vi "Allocate Staff.vi"(0 "Room Service Monitor Model in":refnum<class "Room Service Monitor Model.lvclass">, 5 "Staff Name":string[](array[string]), 11 "error in (no error)":errorcluster) -> (4 "Room Service Monitor Model out":refnum<class "Room Service Monitor Model.lvclass">, 15 "error out":errorcluster)   [LabVIEW 2023, in "Room Service Monitor Model.lvlib" / "Room Service Monitor Model.lvclass"]
uses:
  Room Service Monitor Model.lvclass
  C:/Program Files/National Instruments/LabVIEW 2023/vi.lib/ActorFramework/Actor/Actor.lvclass
  <vilib>/ActorFramework/Actor/Actor.lvclass/Actor.ctl
  <vilib>/ActorFramework/Message Enqueuer/Message Enqueuer.lvclass/Message Enqueuer.ctl
  Room Service Monitor Model.lvclass/Room Service Monitor Model.ctl
  Room Service Monitor Model Messages/Launch Service Monitor Msg/Launch Service Monitor Msg.lvclass/Launch Service Monitor Msg.ctl
  Interfaces/Incoming Hotel Management Tool Model Interface Messages/Update Staff Allocation Msg/Update Staff Allocation Msg.lvclass/Update Staff Allocation Msg.ctl
  <vilib>/ActorFramework/Message Enqueuer/Init from Existing Queue.vi
  <vilib>/ActorFramework/Message Enqueuer/Enqueue.vi
  Room Service Monitor Model Messages/Launch Service Monitor Msg/Launch Service Monitor Msg.lvclass
  C:/Program Files/National Instruments/LabVIEW 2023/vi.lib/ActorFramework/Message/Message.lvclass
  Interfaces/Incoming Hotel Management Tool Model Interface Messages/Update Staff Allocation Msg/Update Staff Allocation Msg.lvclass
  Room Service Monitor Model Messages/Check Staff Msg/Check Staff Msg.lvclass
  <vilib>/ActorFramework/Message Priority Queue/Priority Enqueue.vi
  <vilib>/ActorFramework/Message Enqueuer/Message Enqueuer.lvclass
  Room Service Types/Room Service Base/Room Service Base.lvclass
  <vilib>/ActorFramework/Actor/Actor.lvclass
  C:/Users/bhaghyaraj/Trainings/NI Actor Framework/SDLC/Model Base/Model Base/Model Base.lvclass
  C:/Users/bhaghyaraj/Trainings/NI Actor Framework/SDLC/Interfaces/Model Base/Incoming Model Base Interface.lvclass
  C:/Users/bhaghyaraj/Trainings/NI Actor Framework/SDLC/Room Service Monitor Model/Room Service Monitor Model/Room Service Monitor Model.lvclass
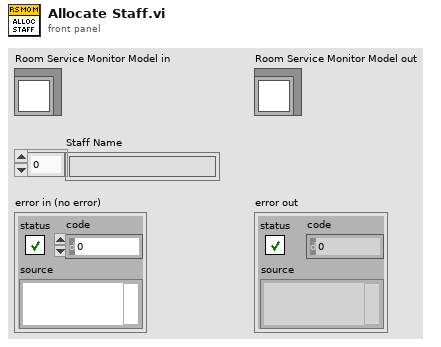
[diagram p1: front panel]
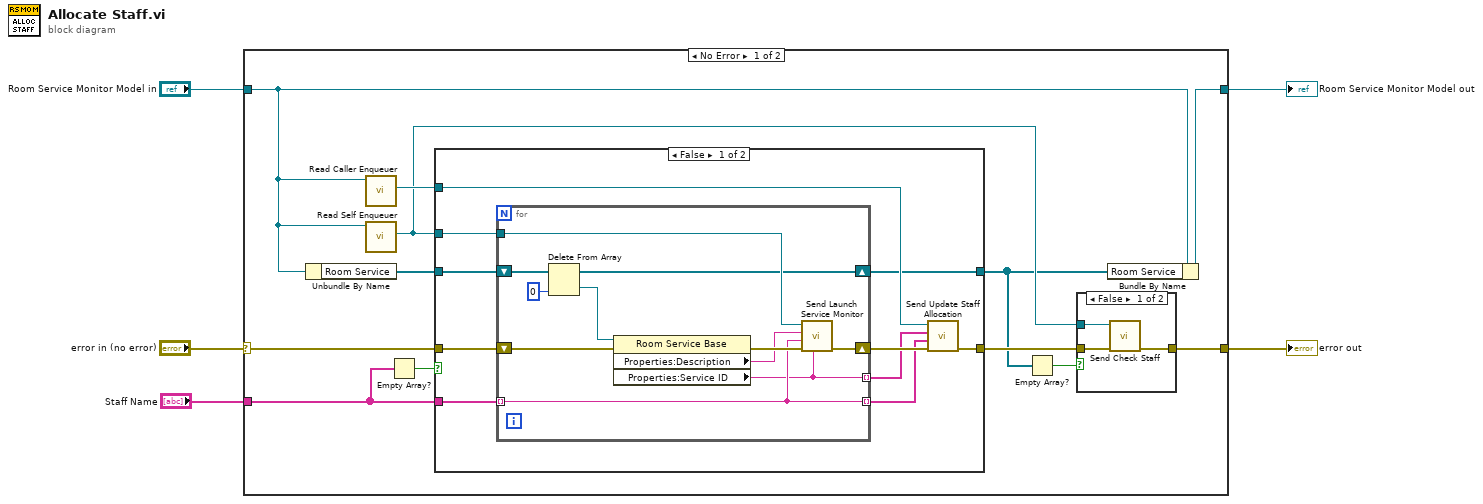
[diagram p0: block diagram]
diagram:
  n1 = case shown="No Error" "error in (no error)" {
    selector: "error in (no error)" -> [w17 w46]
    tunnel: [w8 w46] -> w4
    tunnel: [w11 w45] -> w2
    tunnel: "Room Service Monitor Model in" -> [w15 w45]
    tunnel: "Staff Name" -> [w13 _]
    frame No Error {
      n2 = Unbundle By Name(w15) -> ("Room Service"=w12:refnum<class "Room Service Base.lvclass">[])
      n3 = call <vilib>:"Read Caller Enqueuer.vi"("Actor"=w15) -> ("Caller Enqueuer"=w14:refnum<class "Message Enqueuer.lvclass">)  [unwired: 10 in]
      n4 = call <vilib>:"Read Self Enqueuer.vi"("Actor"=w15) -> ("Self Enqueuer"=w10:refnum<class "Message Enqueuer.lvclass">)  [unwired: 10 in]
      n5 = Empty Array?(array=w13) -> (empty?=w16:bool)
      n6 = case shown="False" w16 {
        tunnel: w17 -> [w27 w43]
        tunnel: [w31 w43] -> w9
        tunnel: w10 -> [w23 _]
        tunnel: w14 -> [w30 _]
        tunnel: w13 -> [w29 _]
        tunnel: w12 -> [w28 w44]
        tunnel: [w22 w44] -> w7
        frame False {
          n7 = for {
            tunnel: w29 -> [w37] mode=indexing
            shift-right: [w40] -> w26
            shift-left: w27 -> [w42]
            tunnel: [w36] -> w25 mode=indexing
            tunnel: [w37] -> w24 mode=indexing
            tunnel: w23 -> [w39]
            shift-right: [w34] -> w22
            shift-left: w28 -> [w35]
            n8 = Delete From Array(array=w35, index=0) -> (deleted portion=w33:refnum<class "Room Service Base.lvclass">, array with subset deleted=w34:refnum<class "Room Service Base.lvclass">[])  [unwired: 1 in]
            n9 = property class="Room Service Base"(reference=w33, error in=w42) -> (error out=w41:errorcluster, "Properties:Description"=w38:string, "Properties:Service ID"=w36:string)  [unwired: 1 out]
            n10 = call "Send Launch Service Monitor.vi"("Service ID"=w36, "error in (no error)"=w41, "Staff Name"=w37, "Description"=w38, "Message Enqueuer"=w39) -> ("error out"=w40:errorcluster)  [unwired: 5 in, 1 out]
          }
          n11 = call "Send Update Staff Allocation.vi"("error in (no error)"=w26, "Staff Name"=w24, "Service ID"=w25, "Message Enqueuer"=w30) -> ("error out"=w31:errorcluster)  [unwired: 6 in, 1 out]
        }
        frame True {
        }
      }
      n12 = Empty Array?(array=w7) -> (empty?=w6:bool)
      n13 = case shown="False" w6 {
        tunnel: w10 -> [w20 _]
        tunnel: w9 -> [w19 w21]
        tunnel: [w18 w21] -> w8
        frame False {
          n14 = call "Send Check Staff.vi"("error in (no error)"=w19, "Message Enqueuer"=w20) -> ("error out"=w18:errorcluster)  [unwired: 8 in, 1 out]
        }
        frame True {
        }
      }
      n15 = Bundle By Name(cluster=w15, "Room Service"=w7) -> (w11:refnum<class "Room Service Monitor Model.lvclass">)
    }
    frame Error {
    }
  }
  "error out" <- w4
  "Room Service Monitor Model out" <- w2
